vi "Untitled 1.vi"() -> ()   [LabVIEW 2016]
panel:
  out "voltage":dbl
  out "voltage Chart 2":dbl(graph)
  in  "mode (CRLF)":T1(ring)=enum."CRLF"
  in  "stop":bool
  out "freq Chart":dbl(graph)
  out "freq":dbl
  in  "address":string
  # "192.168.1.45"
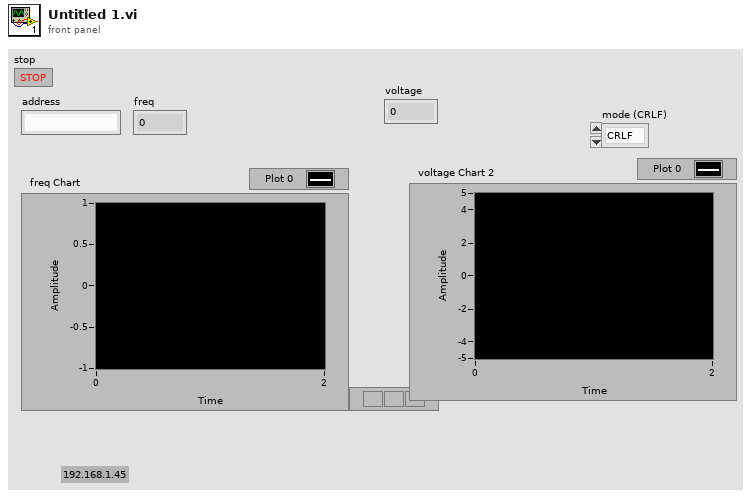
[diagram p1: front panel]
types:
  T1 = enum16{"Standard", "Buffered", "CRLF", "Immediate"}
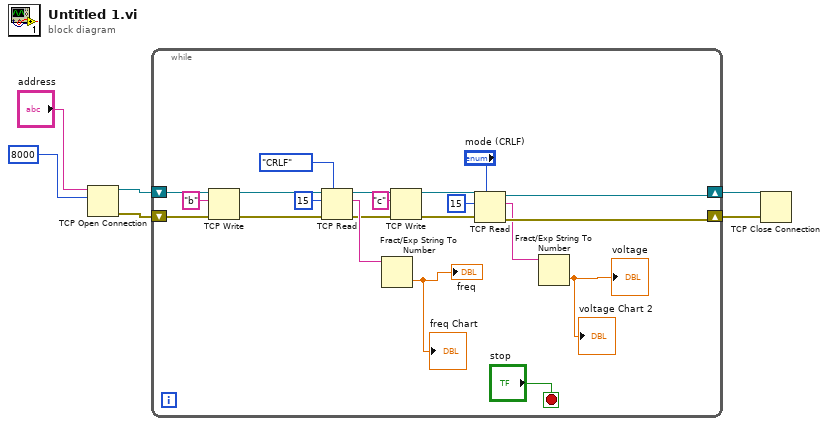
[diagram p0: block diagram]
diagram:
  n1 = TCP Open Connection(address="address", remote port or service name=u16 8000) -> (connection ID=w4:refnum<k5>, error out=w3:errorcluster)  [unwired: 3 in]
  n2 = while {
    shift-right: [w13] -> w2
    shift-left: w4 -> [w27]
    shift-right: [w12] -> w1
    shift-left: w3 -> [w26]
    stop <- "stop" stop-if-true
    n3 = TCP Write(connection ID=w27, data in="b", error in (no error)=w26) -> (connection ID out=w25:refnum<k5>, error out=w24:errorcluster)  [unwired: 1 in, 1 out]
    n4 = TCP Read(connection ID=w25, bytes to read=15, error in (no error)=w24, 7:T1."CRLF" ("mode (standard)")) -> (connection ID out=w17:refnum<k5>, data out=w20:string, error out=w16:errorcluster)  [unwired: 1 in]
    n5 = Fract/Exp String To Number(string=w20) -> (number=→"freq" →"freq Chart":dbl)  [unwired: 3 in, 1 out]
    n6 = TCP Write(connection ID=w17, data in="c", error in (no error)=w16) -> (connection ID out=w15:refnum<k5>, error out=w14:errorcluster)  [unwired: 1 in, 1 out]
    n7 = TCP Read(connection ID=w15, bytes to read=15, error in (no error)=w14, 7:"mode (CRLF)") -> (connection ID out=w13:refnum<k5>, data out=w8:string, error out=w12:errorcluster)  [unwired: 1 in]
    n8 = Fract/Exp String To Number(string=w8) -> (number=→"voltage Chart 2" →"voltage":dbl)  [unwired: 3 in, 1 out]
  }
  n9 = TCP Close Connection(connection ID=w2, error in (no error)=w1) -> ()  [unwired: 1 in, 2 out]
